vi "vna configure.vi"(8 "error in (no error)":errorcluster, 10 "vna settings":T1, 11 "VISA resource name":refnum<visa-resource-name>) -> (0 "error out":errorcluster, 3 "VISA resource name":refnum<visa-resource-name>)   [LabVIEW 2013]
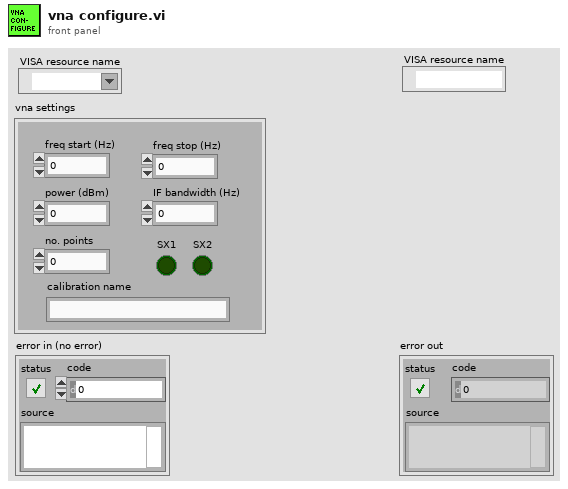
[diagram p1: front panel]
types:
  T1 = cluster{"freq start (Hz)":dbl, "freq stop (Hz)":dbl, "power (dBm)":i32, "IF bandwidth (Hz)":dbl, "no. points":i32, "calibration name":string, "SX1":bool, "SX2":bool}
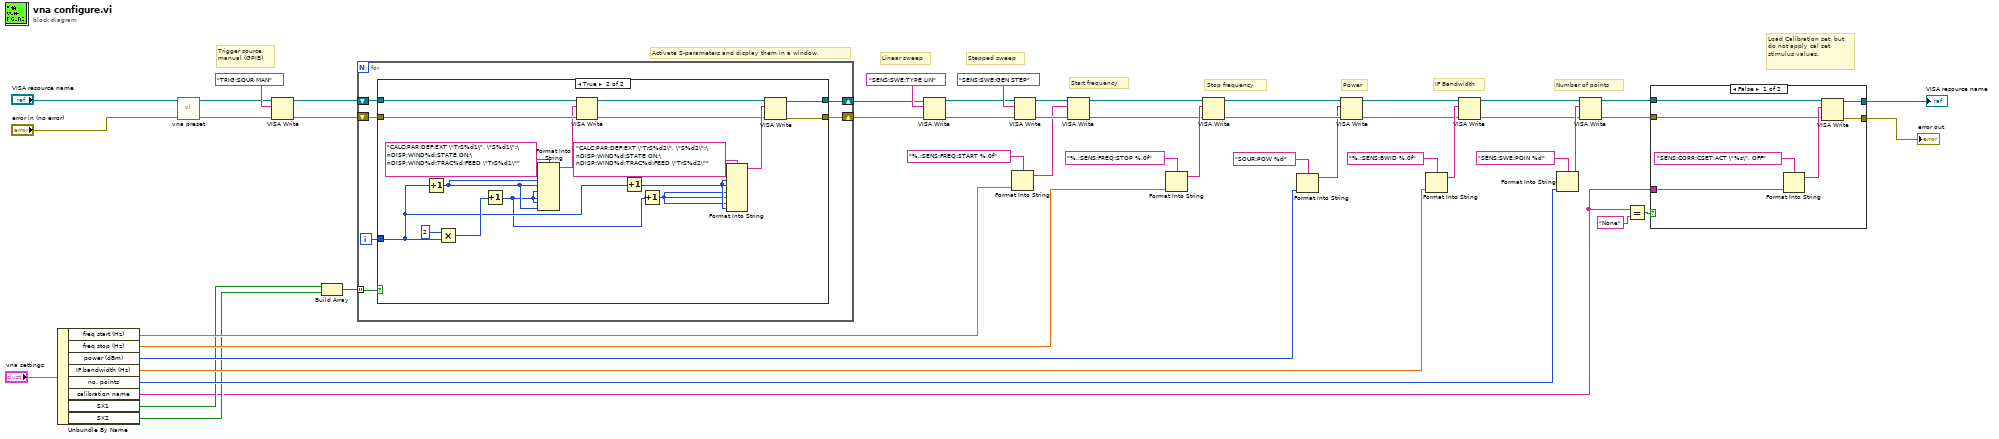
[diagram p0: block diagram]
diagram:
  # "Activate S-parameters and display them in a window."
  # "Load Calibration set, but do not apply cal set stimulus values."
  # "Number of points"
  # "IF Bandwidth"
  # "Power"
  # "Stop frequency"
  # "Start frequency"
  # "Stepped sweep"
  # "Linear sweep"
  # "Trigger source \nmanual (GPIB)"
  n1 = Unbundle By Name("vna settings") -> ("freq start (Hz)"=w42:dbl, "freq stop (Hz)"=w37:dbl, "power (dBm)"=w32:i32, "IF bandwidth (Hz)"=w27:dbl, "no. points"=w22:i32, "calibration name"=w1:string, "SX1"=w17:bool, "SX2"=w16:bool)
  n2 = call "vna preset.vi"("error in (no error)"="error in (no error)", "VISA resource name"="VISA resource name") -> ("error out"=w11:errorcluster, "VISA resource name 2"=w10:refnum<visa-resource-name>)  [unwired: 8 in]
  n3 = VISA Write(VISA resource name=w10, write buffer="TRIG:SOUR MAN", error in (no error)=w11) -> (VISA resource name out=w15:refnum<visa-resource-name>, error out=w14:errorcluster)  [unwired: 1 out]
  n4 = Build Array(w17, w16) -> (w18:bool[])
  n5 = for {
    tunnel: w18 -> [w55] mode=indexing
    shift-right: [w52] -> w13
    shift-left: w15 -> [w54]
    shift-right: [w51] -> w12
    shift-left: w14 -> [w53]
    i -> [w50]
    n6 = case shown="True" w55 {
      tunnel: w54 -> [w57 w73]
      tunnel: [w57 w65] -> w52
      tunnel: w53 -> [w56 w72]
      tunnel: [w56 w66] -> w51
      tunnel: w50 -> [_ w62]
      frame False {
      }
      frame True {
        n7 = Increment(x=w62) -> (x+1=w61:i32)
        n8 = Multiply(x=2, y=w62) -> (x*y=w63:i32)
        n9 = Increment(x=w63) -> (x+1=w60:i32)
        n10 = Format Into String(format string="CALC:PAR:DEF:EXT \"TrS%d1\", \"S%d1\";\nDISP:WIND%d:STATE ON;\nDISP:WIND%d:TRAC%d:FEED \"TrS%d1\"", w61, w61, w60, w60, w60, w61) -> (resulting string=w71:string)  [unwired: 2 in, 1 out]
        n11 = VISA Write(VISA resource name=w73, write buffer=w71, error in (no error)=w72) -> (VISA resource name out=w68:refnum<visa-resource-name>, error out=w67:errorcluster)  [unwired: 1 out]
        n12 = Increment(x=w62) -> (x+1=w59:i32)
        n13 = Increment(x=w60) -> (x+1=w58:i32)
        n14 = Format Into String(format string="CALC:PAR:DEF:EXT \"TrS%d2\", \"S%d2\";\nDISP:WIND%d:STATE ON;\nDISP:WIND%d:TRAC%d:FEED \"TrS%d2\"", w59, w59, w58, w58, w58, w59) -> (resulting string=w69:string)  [unwired: 2 in, 1 out]
        n15 = VISA Write(VISA resource name=w68, write buffer=w69, error in (no error)=w67) -> (VISA resource name out=w65:refnum<visa-resource-name>, error out=w66:errorcluster)  [unwired: 1 out]
      }
    }
  }
  n16 = VISA Write(VISA resource name=w13, write buffer="SENS:SWE:TYPE LIN", error in (no error)=w12) -> (VISA resource name out=w45:refnum<visa-resource-name>, error out=w44:errorcluster)  [unwired: 1 out]
  n17 = Format Into String(format string="%.;SENS:FREQ:START %.0f", w42) -> (resulting string=w39:string)  [unwired: 2 in, 1 out]
  n18 = VISA Write(VISA resource name=w45, write buffer="SENS:SWE:GEN STEP", error in (no error)=w44) -> (VISA resource name out=w41:refnum<visa-resource-name>, error out=w40:errorcluster)  [unwired: 1 out]
  n19 = VISA Write(VISA resource name=w41, write buffer=w39, error in (no error)=w40) -> (VISA resource name out=w35:refnum<visa-resource-name>, error out=w34:errorcluster)  [unwired: 1 out]
  n20 = Format Into String(format string="%.;SENS:FREQ:STOP %.0f", w37) -> (resulting string=w36:string)  [unwired: 2 in, 1 out]
  n21 = VISA Write(VISA resource name=w35, write buffer=w36, error in (no error)=w34) -> (VISA resource name out=w30:refnum<visa-resource-name>, error out=w31:errorcluster)  [unwired: 1 out]
  n22 = Format Into String(format string="SOUR:POW %d", w32) -> (resulting string=w29:string)  [unwired: 2 in, 1 out]
  n23 = VISA Write(VISA resource name=w30, write buffer=w29, error in (no error)=w31) -> (VISA resource name out=w24:refnum<visa-resource-name>, error out=w25:errorcluster)  [unwired: 1 out]
  n24 = Format Into String(format string="%.;SENS:BWID %.0f", w27) -> (resulting string=w26:string)  [unwired: 2 in, 1 out]
  n25 = VISA Write(VISA resource name=w24, write buffer=w26, error in (no error)=w25) -> (VISA resource name out=w20:refnum<visa-resource-name>, error out=w19:errorcluster)  [unwired: 1 out]
  n26 = Format Into String(format string="SENS:SWE:POIN %d", w22) -> (resulting string=w21:string)  [unwired: 2 in, 1 out]
  n27 = VISA Write(VISA resource name=w20, write buffer=w21, error in (no error)=w19) -> (VISA resource name out=w6:refnum<visa-resource-name>, error out=w7:errorcluster)  [unwired: 1 out]
  n28 = Equal?(x=w1, y="None") -> (x = y?=w2:bool)
  n29 = case shown="False" w2 {
    tunnel: w7 -> [w79 w82]
    tunnel: w6 -> [w78 w83]
    tunnel: [w77 w83] -> w5
    tunnel: [w76 w82] -> w4
    tunnel: w1 -> [w75 _]
    frame False {
      n30 = Format Into String(format string="SENS:CORR:CSET:ACT \"%s\", OFF", w75) -> (resulting string=w81:string)  [unwired: 2 in, 1 out]
      n31 = VISA Write(VISA resource name=w78, write buffer=w81, error in (no error)=w79) -> (VISA resource name out=w77:refnum<visa-resource-name>, error out=w76:errorcluster)  [unwired: 1 out]
    }
    frame True {
    }
  }
  "VISA resource name" <- w5
  "error out" <- w4
